vi "write exception property.vi"   [LabVIEW 2013, in "Write Variant Repository.xnode"]
doc: "This VI is used to store data similar to a look up table, into a Variant data type. This VI is will set an attribute of the <b>Variant Repository In</b>, with the tag name of <b>Tag</b>, value of <b>Value</b>, and then return the new <b>Varient Repository Out</b>. This VI will also return whether or not the new tag being written is replacing an old one or not, in the <b>Replaced?</b> boolean.\n\nThe tag name it self is optional and if one is not provided then the label name on the <b>Value</b> data will be used.\n\nOptionally the <b>Write Once?</b> boolean can be used. If true this will generate an error, if the tag that is trying to be written is already written. In this way the tag can only be written once without generating an error. By default this is set to false.\n\nTo read multiple tags right click and choose Read Multiple Tags.\n\n-------------\nBrian Hoover (Hooovahh)\n\nProduct Name: Variant Repository\nPackage File Name: lava_lib_variant_repository\nPackage Version: 1.0.1.11\nMinimum LabVIEW Version: 11.0"
uses:
  Write Variant Repository/Write Variant Repository.xnode
  severity.ctl
  exception.lvlib
  category.ctl
  exception.ctl
  Write Variant Repository/Write Exception Property.xnode
  <vilib>/Utility/VariantDataType/GetTypeInfo.vi
  <vilib>/Utility/VariantDataType/VariantType.lvlib
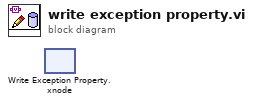
[diagram p0: block diagram]
diagram:
  n1 = xnode "Write Exception Property.xnode"() -> ()  [unwired: 4 in, 3 out]
